vi "Collect Signal on Datavalid.vi"(9 "Data Valid":bool, 10 "Input":dbl) -> (2 "Output":dbl[](array[numeric]) format="%.2f")   [LabVIEW 2012]
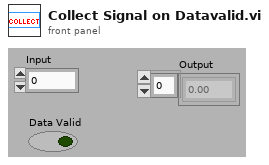
[diagram p1: front panel]
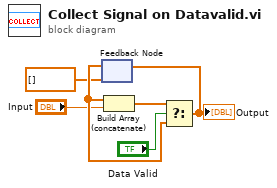
[diagram p0: block diagram]
diagram:
  n1 = feedback #1(dbl[] []) -> (w4:dbl[])
  n2 = Build Array (concatenate)(w4, "Input") -> (w6:dbl[])
  n3 = Select(t=w6, s="Data Valid", f=w4) -> (s? t:f=w5:dbl[])
  "Output" <- w5
  n4 = feedback-in #1(w5) -> ()
